vi "Destroy Error Queue.vi"(8 "error in (no error)":errorcluster, 11 "Error Queue":T1) -> (0 "error out":errorcluster, 2 "remaining errors":errorcluster[](array[cluster]))   [LabVIEW 2017, in "Data Sharing Framework Engine.lvlib" / "Engine Interface.lvclass"]
uses:
  Engine Interface.lvclass
  Error Queue Ref.ctl
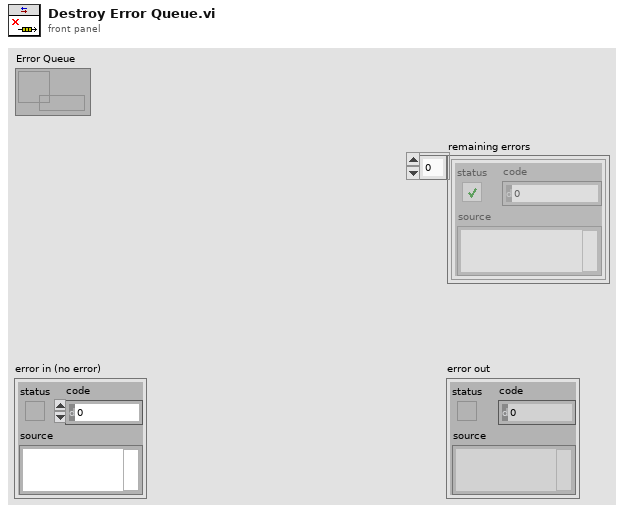
[diagram p1: front panel]
types:
  T1 = typedef "Data Sharing Framework Engine.lvlib/Engine Interface.lvclass/Error Queue Ref.ctl" = refnum<queue>
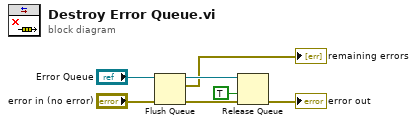
[diagram p0: block diagram]
diagram:
  n1 = Flush Queue(queue="Error Queue", error in (no error)="error in (no error)") -> (queue out=w5:T1, remaining elements=→"remaining errors":errorcluster[], error out=w3:errorcluster)
  n2 = Release Queue(queue=w5, force destroy? (F)=TRUE, error in (no error)=w3) -> (error out=→"error out":errorcluster)  [unwired: 2 out]
